vi "300 lbs Tension.vi"() -> ()   [LabVIEW 2013]
uses:
  <vilib>/Analysis/baseanly.llb/Mean (DBL).vi
  Instance           1 34Saved   TDCB-Multiplot-With-Unload .vi
  Instance           2 34Saved   TDCB-Multiplot-With-Unload .vi
  <vilib>/Analysis/NI_AALBase.lvlib
panel:
  out "Crosshead Displacement":cluster{dbl[], dbl[]}(graph)
  in  "Unload Velocity":dbl=500.0
  in  "Load Cell\nSelection":enum16{"300lb", "5lb", "50lb", "100lb"}(ring)
  in  "Distance to Travel (microns) \nup is positive":dbl=250000.0
  in  "Velocity (microns/sec)":dbl=10.0
  in  "Unload":bool
  in  "Filename":string
  in  "Storage Directory":path=path "D:/AMS_Users_2014_2015/Michael Rossol"
  in  "Material":string
  in  "Stop":bool
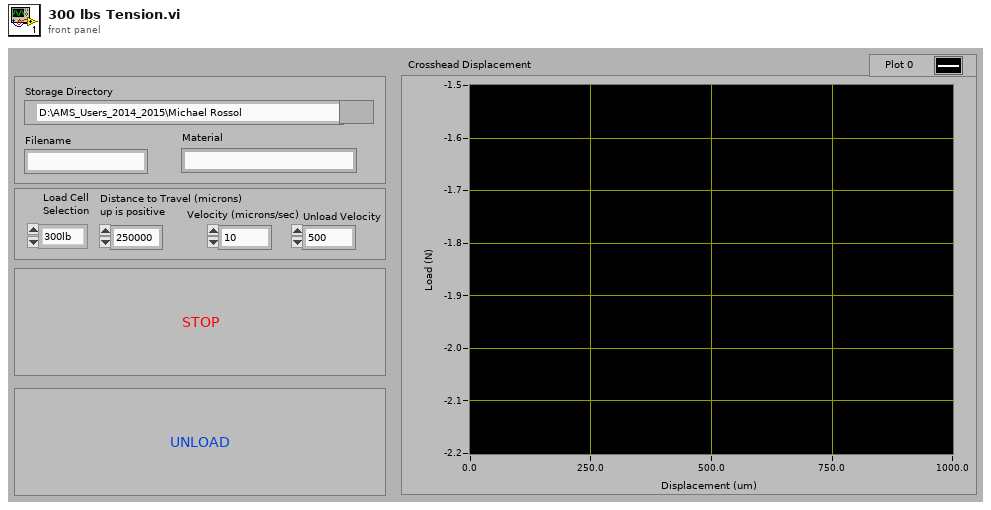
[diagram p1: front panel]
types:
  T1 = enum16{"open", "open or create", "create or replace", "create", "open (read only)"}
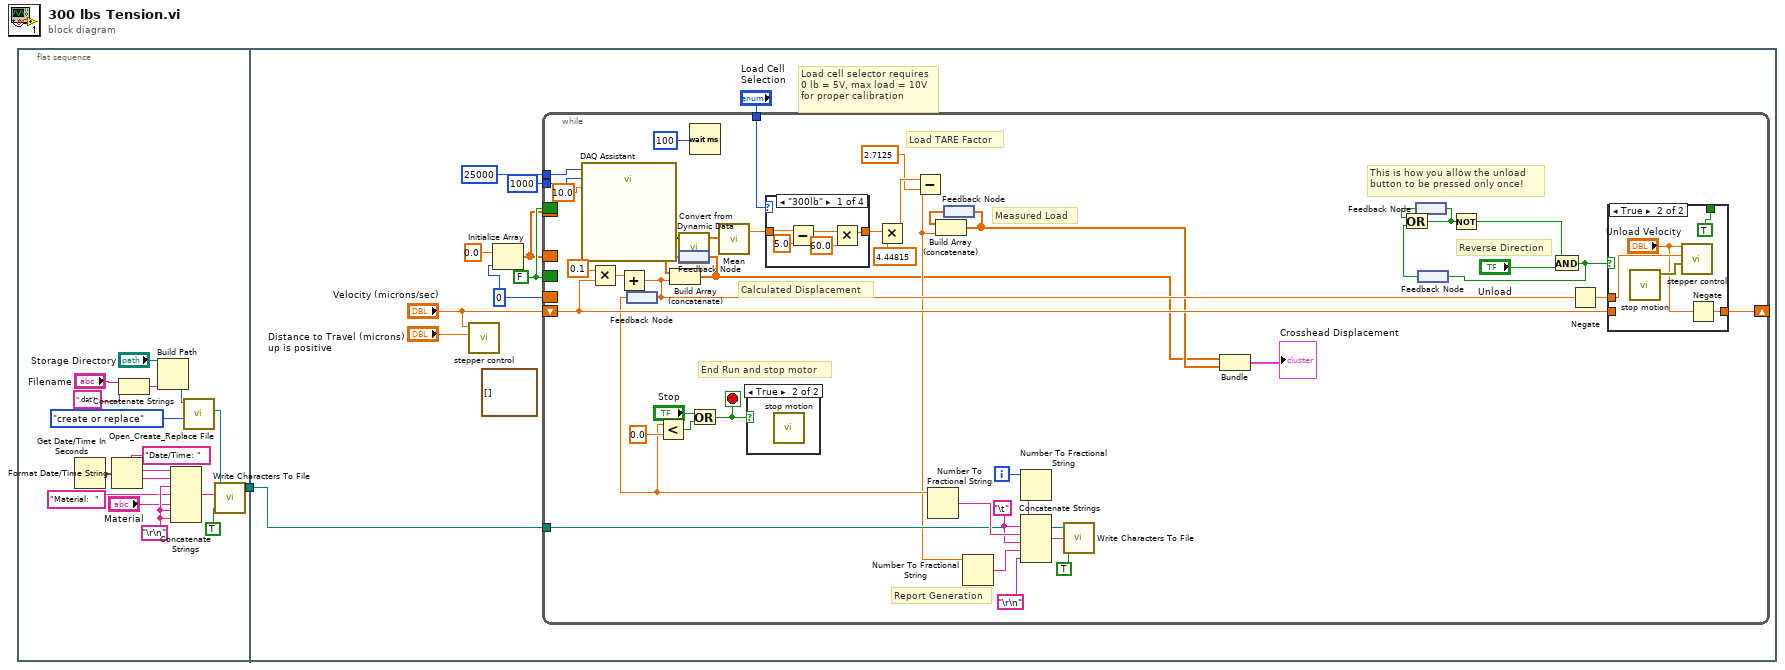
[diagram p0: block diagram]
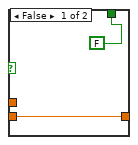
[diagram p2: hidden frame]
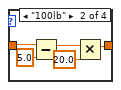
[diagram p4: hidden frame]
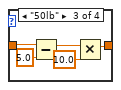
[diagram p5: hidden frame]
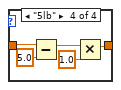
[diagram p6: hidden frame]
diagram:
  n1 = flat-sequence {
    tunnel: [w2] -> w1
    tunnel: w1 -> [w18]
    frame #0 {
      w13 = "\r\n"
      n2 = Get Date/Time In Seconds() -> (seconds since 1Jan1904=w14:timestamp)
      n3 = Format Date/Time String(seconds (now)=w14) -> (date/time string=w4:string)  [unwired: 2 in]
      n4 = Concatenate Strings("Filename", ".dat") -> (w10:string)
      n5 = Build Path(base path="Storage Directory", name or relative path=w10) -> (appended path=w15:path)
      n6 = Concatenate Strings("Date/Time: ", w4, w13, "Material:  ", "Material", w13, w13) -> (w7:string)
      n7 = call <vilib>:"Open_Create_Replace File.vi"("function (open:0)"=T1."create or replace", "file path"=w15) -> ("new file path"=w16:path)  [unwired: 6 in, 3 out]
      n8 = call <vilib>:"Write Characters To File.vi"("append to file? (new file:F)"=TRUE, "character string"=w7, "file path (dialog if empty)"=w16) -> ("new file path (Not A Path if cancelled)"=w2:path)  [unwired: 2 in]
    }
    frame #1 {
      w27 = FALSE
      (unwired) cluster{"slope":dbl, "intercept":dbl}[] []
      w26 = 0 ("dimension size")
      # "Load cell selector requires\n0 lb = 5V, max load = 10V\nfor proper calibration"
      n9 = call "stepper control.vi"("Distance to Travel (microns) \nup  is positive"="Distance to Travel (microns) \nup is positive", "Velocity (microns/sec)"="Velocity (microns/sec)") -> ()  [unwired: 9 in, 1 out]
      n10 = Initialize Array(0.0 ("element"), w26) -> (w25:dbl[])
      n11 = while {
        tunnel: 25000 ("Sampling Rate") -> [w71]
        tunnel: 1000 ("Samples") -> [w70]
        tunnel: "Load Cell\nSelection" -> [w66]
        tunnel: w18 -> [w52]
        shift-right: [w48] -> _
        shift-left: "Velocity (microns/sec)" -> [w47]
        border: w25 -> [_]
        border: w26 -> [_]
        border: w25 -> [_]
        border: w27 -> [_]
        border: w27 -> [_]
        i -> [w51]
        stop <- w46 stop-if-true
        w53 = "\t"
        # "Load TARE Factor"
        # "This is how you allow the unload\nbutton to be pressed only once!"
        # "Reverse Direction"
        # "Calculated Displacement"
        # "Measured Load"
        # "End Run and stop motor"
        # "Report Generation"
        n12 = call "DAQ Assistant"("rate"=w71, "number of samples"=w70, "timeout (s)"=10.0 ("timeout (sec)")) -> ("data"=w68:dynamicdata)  [unwired: 14 in, 2 out]
        n13 = Multiply(x=0.1, y=w47) -> (x*y=w43:dbl)
        n14 = feedback #1() -> (w42:dbl)
        n15 = Add(x=w43, y=w42) -> (x+y=w50:dbl)
        n16 = feedback-in #1(w50) -> ()
        n17 = Less?(x=w42, y=0.0) -> (x < y?=w45:bool)
        n18 = call "Convert from Dynamic Data"("Dynamic Data Type"=w68) -> ("Array"=w67:dbl[])  [unwired: 3 in]
        n19 = feedback #2() -> (w61:dbl[])
        n20 = Build Array (concatenate)(w61, w50) -> (w28:dbl[])
        n21 = feedback-in #2(w28) -> ()
        n22 = Wait (ms)(milliseconds to wait=100 ("Loop Timing")) -> ()  [unwired: 1 out]
        n23 = Or(x="Stop", y=w45) -> (x .or. y?=w46:bool)
        n24 = call-poly <vilib>:"Mean.vi"("X"=w67) -> ("mean"=w65:dbl)  [unwired: 1 out]
        n25 = case shown="True" w46 {
          frame False {
          }
          frame True {
            n26 = call "stop motion.vi"() -> ()  [unwired: 11 in, 1 out]
          }
        }
        n27 = case shown="\"300lb\"" w66 {
          tunnel: w65 -> [w80 w85 w93 w98]
          tunnel: [w79 w84 w92 w97] -> w63
          frame "300lb" {
            n28 = Subtract(x=w80, y=5.0) -> (x-y=w82:dbl)
            n29 = Multiply(x=w82, y=60.0) -> (x*y=w79:dbl)
          }
          frame "100lb" {
            n30 = Subtract(x=w85, y=5.0) -> (x-y=w87:dbl)
            n31 = Multiply(x=w87, y=20.0) -> (x*y=w84:dbl)
          }
          frame "50lb" {
            n32 = Subtract(x=w93, y=5.0) -> (x-y=w90:dbl)
            n33 = Multiply(x=w90, y=10.0) -> (x*y=w92:dbl)
          }
          frame "5lb" {
            n34 = Subtract(x=w98, y=5.0) -> (x-y=w95:dbl)
            n35 = Multiply(x=w95, y=1.0) -> (x*y=w97:dbl)
          }
        }
        n36 = Multiply(x=w63, y=4.44815) -> (x*y=w33:dbl)
        n37 = Subtract(x=w33, y=2.7125) -> (x-y=w32:dbl)
        n38 = Number To Fractional String(number=w42) -> (F-format string=w56:string)  [unwired: 3 in]
        n39 = feedback #3() -> (w62:dbl[])
        n40 = Build Array (concatenate)(w62, w32) -> (w29:dbl[])
        n41 = feedback-in #3(w29) -> ()
        n42 = Number To Fractional String(number=w32) -> (F-format string=w54:string)  [unwired: 3 in]
        n43 = Number To Fractional String(number=w51) -> (F-format string=w59:string)  [unwired: 3 in]
        n44 = Concatenate Strings(w59, w53, w56, w53, w54, "\r\n") -> (w58:string)
        n45 = call <vilib>:"Write Characters To File.vi"("append to file? (new file:F)"=TRUE, "character string"=w58, "file path (dialog if empty)"=w52) -> ()  [unwired: 2 in, 1 out]
        n46 = Bundle(w28, w29) -> (→"Crosshead Displacement":cluster{dbl[], dbl[]})  [unwired: 1 in]
        n47 = feedback #4() -> (w41:bool)
        n48 = feedback #5() -> (w38:bool)
        n49 = Or(x=w41, y=w38) -> (x .or. y?=w40:bool)
        n50 = feedback-in #4(w40) -> ()
        n51 = Not(x=w40) -> (.not. x?=w39:bool)
        n52 = And(x=w39, y="Unload") -> (x .and. y?=w36:bool)
        n53 = feedback-in #5(w36) -> ()
        n54 = Negate(x=w50) -> (-x=w49:dbl)
        n55 = case shown="True" w36 {
          tunnel: w49 -> [_ w77]
          tunnel: [w73 w76] -> w48
          tunnel: w47 -> [w73 _]
          tunnel: [FALSE TRUE] -> _
          frame False {
          }
          frame True {
            n56 = call "stop motion.vi"() -> ("error out"=w78:errorcluster)  [unwired: 11 in]
            n57 = call "stepper control.vi"("error in (no error)"=w78, "Distance to Travel (microns) \nup  is positive"=w77, "Velocity (microns/sec)"="Unload Velocity") -> ()  [unwired: 8 in, 1 out]
            n58 = Negate(x="Unload Velocity") -> (-x=w76:dbl)
          }
        }
      }
    }
  }
